vi "Measure Loop Period.vi"(8 "error in (no error)":errorcluster, 11 "PID Loop in":refnum<class "PID Loop.lvclass">) -> (0 "error out":errorcluster, 2 "dt":dbl, 3 "PID Loop out":refnum<class "PID Loop.lvclass">)   [LabVIEW 2024, in "PID Loop.lvlib" / "PID Loop.lvclass"]
uses:
  PID Loop.lvclass
  PID Loop.lvclass/PID Loop.ctl
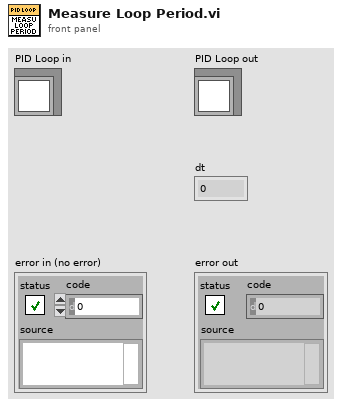
[diagram p1: front panel]
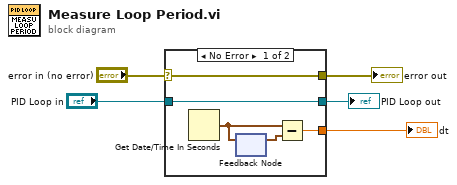
[diagram p0: block diagram]
diagram:
  n1 = case shown="No Error" "error in (no error)" {
    selector: "error in (no error)" -> [w9 w12]
    tunnel: [w9 w12] -> w4
    tunnel: [w10 w11] -> w2
    tunnel: "PID Loop in" -> [w10 w11]
    tunnel: [w6 _] -> w1
    frame No Error {
      n2 = Get Date/Time In Seconds() -> (seconds since 1Jan1904=w8:timestamp)
      n3 = feedback-in #1(w8) -> ()
      n4 = feedback #1() -> (w7:timestamp)  [unwired: 1 in]
      n5 = Subtract(x=w8, y=w7) -> (x-y=w6:dbl)
    }
    frame Error {
    }
  }
  "error out" <- w4
  "PID Loop out" <- w2
  "dt" <- w1
